vi "FGV - Authorization Data.vi"(6 "State - FGV":T1=enum."Read", 8 "Error In":errorcluster, 11 "Data In":string[][](array[string])) -> (0 "Error Out":errorcluster, 3 "Data Out":string[][](array[string]))   [LabVIEW 2020]
uses:
  Control/State - FGV.ctl
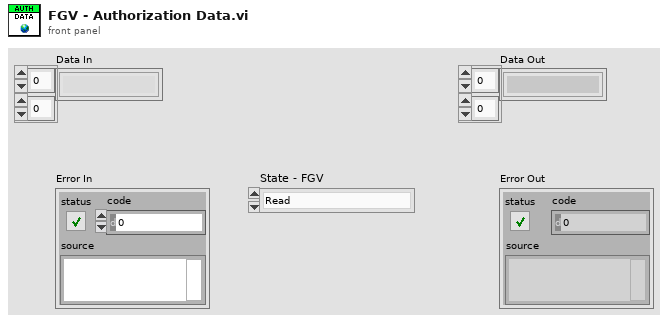
[diagram p1: front panel]
types:
  T1 = typedef "State - FGV.ctl" = enum16{"Write", "Read"}
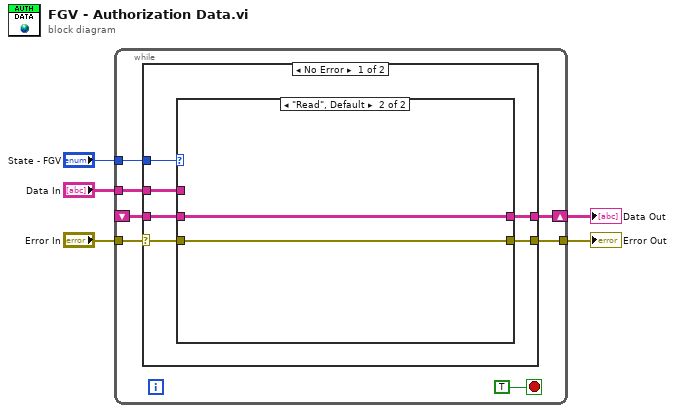
[diagram p0: block diagram]
diagram:
  n1 = while {
    tunnel: "Error In" -> [w12]
    tunnel: [w11] -> w4
    tunnel: "State - FGV" -> [w9]
    shift-right: [w6] -> w2
    shift-left: _ -> [w8]
    tunnel: "Data In" -> [w7]
    stop <- TRUE stop-if-true
    n2 = case shown="No Error" w12 {
      selector: w12 -> [w18 w24]
      tunnel: [w17 w24] -> w11
      tunnel: w9 -> [w16 _]
      tunnel: w8 -> [w15 w23]
      tunnel: w7 -> [w14 _]
      tunnel: [w13 w23] -> w6
      frame No Error {
        n3 = case shown="\"Read\", Default" w16 {
          tunnel: w18 -> [w20 w22]
          tunnel: [w20 w22] -> w17
          tunnel: w15 -> [_ w21]
          tunnel: w14 -> [w19 _]
          tunnel: [w19 w21] -> w13
          frame "Write" {
          }
          frame "Read", Default {
          }
        }
      }
      frame Error {
      }
    }
  }
  "Error Out" <- w4
  "Data Out" <- w2
